vi "TSCANFD_SetData_Regs.vi"(8 "ERROR IN":errorcluster caption="错误输入（无错误）", 9 "AppName":string="LABFD", 10 "CANFD_Config_Regs":T1={"CANFD Configuration"={"Hardware Type"=8, "Hardware Subtype"=enum."TC1016", "AArbRateKbps"=250.0, "AListenOnly"=enum."Normal", "Int120Ohm"=enum."Enable", "EnableChannel"=enum."Enable", "AHwChannel"=0, "AAppChannel"=0, "ADataRateKbps"=250.0, "AControllerType"=0, "AControllerMode"=0, "AldHW"=0}, "CANFD_Sampling point"={"AArbSEG1"=0, "AArbSEG2"=0, "AArbPrescaler"=0, "AArbSJW"=0, "ADataSEG1"=0, "ADataSEG2"=0, "ADataPrescaler"=0, "ADataSJW"=0}} {"CANFD Configuration"."Hardware Type" items=["BUS_UNKNOWN_TYPE", "TS_TCP_DEVICE", "XL_USB_DEVICE", "TS_USB_DEVICE", "PEAK_USB_DEVICE", "KVASER_USB_DEVICE", "ZLG_USB_DEVICE", "ICS_USB_DEVICE", "TS_TC1005_DEVICE", "CANABLE_USB_DEVICE", "TS_WIRELESS_OBD", "TS_USB_DEVICE_EX", "IXXAT_USB_DEVICE", "TS_ETH_IF_DEVICE", "TS_USB_IF_DEVICE", "BUS_DEV_TYPE_COUNT"]; "CANFD Configuration"."AHwChannel" items=["CHN1", "CHN2", "CHN3", "CHN4", "CHN5", "CHN6", "CHN7", "CHN8", "CHN9", "CHN10", "CHN11", "CHN12", "CHN13", "CHN14", "CHN15", "CHN16", "CHN17", "CHN18", "CHN19", "CHN20", "CHN21", "CHN22", "CHN23", "CHN24", "CHN25", "CHN26", "CHN27", "CHN28", "CHN29", "CHN30", "CHN31", "CHN32"]; "CANFD Configuration"."AAppChannel" items=["CHN1", "CHN2", "CHN3", "CHN4", "CHN5", "CHN6", "CHN7", "CHN8", "CHN9", "CHN10", "CHN11", "CHN12", "CHN13", "CHN14", "CHN15", "CHN16", "CHN17", "CHN18", "CHN19", "CHN20", "CHN21", "CHN22", "CHN23", "CHN24", "CHN25", "CHN26", "CHN27", "CHN28", "CHN29", "CHN30", "CHN31", "CHN32"]; "CANFD Configuration"."AControllerType" items=["lfdtCAN", "lfdtISOFDCAN", "lfdtNonISOFDFDCAN"]; "CANFD Configuration"."AControllerMode" items=["lfdmNormal", "lfdmACKOff", "lfdmRestricted"]}, 11 "PATH":path) -> (0 "ERROR OUT":errorcluster caption="错误输出", 3 "PATH OUT":path, 4 "configure_baudrate_return":i32, 6 "mapping_return":i32)   [LabVIEW 2014]
doc: "tsapp_set_mapping_verbose ：\nFunction Introduction ：\nBefore using hardware devices, map the channels (CAN/CANFD/LIN) for the application program\n(i.e. binding) specifies the designated channel of the CAN device. This operation can also be performed on\nThe device management interface of TSMaster is completed, and this part of the operation is not required in the code.\nRegarding the channel mapping function, there are still unclear areas. Please refer to the document: TsMasterApi HardwareMap.pdf\nCall location ：\nCall this function to complete the hardware binding before the application connects to the CAN tool.\ninput parameter \nAppName: Application Name: The name of the application bound to this Map, which should be consistent with the name in initialized lib_tsmaster\nagreement\nAAppChannelType: Channel type: including APP_CAN, APP_LIN AAppChannel: Channel number of the application: This is the channel number used by the upper level program\nAHardwareName: Hardware name: such as TOSUN, Vector, etc., can also be left blank, mainly for the convenience of users to view\nAHardwareType: Hardware type: According to TLIBBusToolDeviceType, it includes all mainstream CANs currently on the market\nCard hardware Among them, the definition of tool enumeration types is as follows:\npublic enum TLIBBusToolDeviceType : int {\nBUS_UNKNOWN_TYPE = 0, TS_TCP_DEVICE = 1, XL_USB_DEVICE = 2, TS_USB_DEVICE = 3, PEAK_USB_DEVICE = 4, KVASER_USB_DEVICE = 5, ZLG_USB_DEVICE = 6, ICS_USB_DEVICE = 7, TS_TC1005_DEVICE = 8\n};\nAHardwareSubType: The sub devices under this device type, such as TS-USB-Device on the same star, are included below TC1001, TL1002, TC1011 and other series of products\nAHardwareIndex: Supports inserting multiple identical hardware devices simultaneously, such as inserting two TC1001 devices at the same time. This is used to select\nIs it the channel of device 1 or device 2\nAHardwareChannel: The channel for hardware devices, for example, TC1005 has 5 hardware channels, and this parameter is used to select the appropriate one\nCorresponding hardware channels\nAEnable Mapping: Is this mapping enabled? If set to false, the channel cannot be used。\nReturn value ：\n==0: Execution successful\nOther: Query error code\n\n\ntsapp_configure_baudrate_canfd :\nFunction Name\nint tsapp_configure_baudrate_canfd( int AIdxChn, Single AArbRateKbps, Single ADataRateKbps, TLIBCANFDControllerType AControllerType, TLIBCANFDControllerMode AControllerMode, Boolean AInstallTermResistor120Ohm);\nFunction Introduction\nConfigure hardware parameters such as baud rate for CANFD channel\nCall location\nBefore connecting to the CAN tool, call this function to configure hardware device parameters\n\ninput parameter :\nAIdxChn: Application Channel\nAArbRateKbps: Arbitration field baud rate\nADataRateKbps: Data field baud rate\nACcontrollerType: Controller type, including: Classic CAN (lfdtCAN=0), ISOCANFD (lfdtISOCAN)=\n1) NoISOCANFD (lfdtNonISOCAN=2) ACntrollerMode: Controller working mode, including: normal working mode (lfdmNormal=0), disable ACK mode\n(lfdmaCKOff=1), Restricted Mode (lfdmaRestricted=2) AInstallTermResistor120Ohm: Enable internal terminal resistance\nReturn value :\n==0: Connection successful\nOther: Check for error codes"
uses:
  Utilities/Typedef/Hardware_Subtype.ctl
  Typedef/TSCAN_CANFD_Configuration.ctl
  Typedef/TSCAN_CANFD_Configuration_Regs.ctl
  All_Control/Typedef/Hardware Type.ctl
panel:
  # "用N路can通道，设置N路CAN通道"
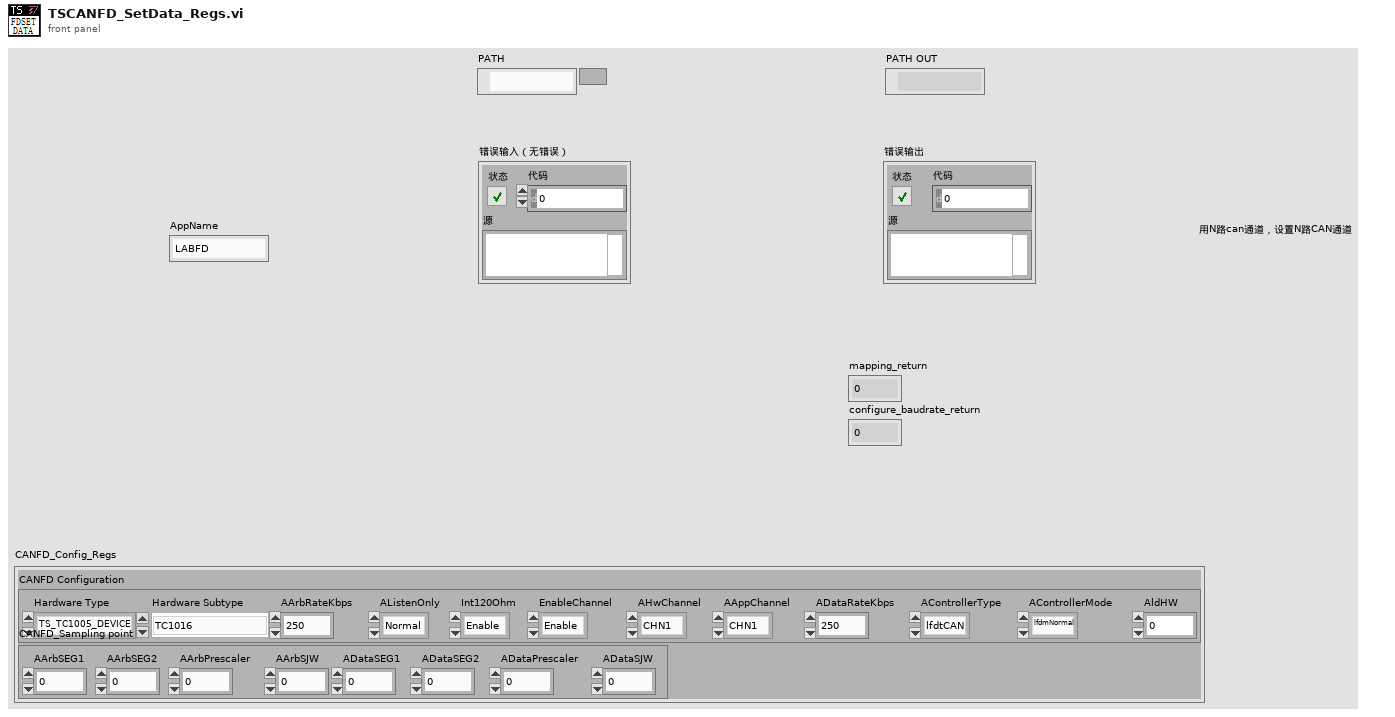
[diagram p1: front panel]
types:
  T1 = typedef "TSCAN_CANFD_Configuration_Regs.ctl" = cluster{"CANFD Configuration":T2, "CANFD_Sampling point":cluster{"AArbSEG1":i32, "AArbSEG2":i32, "AArbPrescaler":i32, "AArbSJW":i32, "ADataSEG1":i32, "ADataSEG2":i32, "ADataPrescaler":i32, "ADataSJW":i32}}
  T2 = typedef "TSCAN_CANFD_Configuration.ctl" = cluster{"Hardware Type":T3, "Hardware Subtype":T4, "AArbRateKbps":sgl, "AListenOnly":enum16{"Normal", "ListenOnly"}, "Int120Ohm":enum16{"Disable", "Enable"}, "EnableChannel":enum16{"Disable", "Enable"}, "AHwChannel":i32, "AAppChannel":i32, "ADataRateKbps":sgl, "AControllerType":i32, "AControllerMode":i32, "AldHW":i32}
  T3 = typedef "Hardware Type.ctl" = i32
  T4 = typedef "Hardware_Subtype.ctl" = enum16{"TS_UNKNOWN_DEVICE", "TSCAN_PRO", "TSCAN_Lite1", "TC1001", "TL1001", "TC1011", "TM5011", "TC1002", "TC1014", "TSCANFD2517", "TC1026", "TC1016", "TC1012", "TC1013", "TLog1002", "TC1034", "TC1018", "GW2116", "TC2115", "MP1013", "TC1113", "TC1114", "TP1013", "TC1017", "TP1018", "TF10XX", "TL1004_FD_4_LIN_2", "TE1051", "TP1051", "TP1034", "TTS9015", "TP1026", "TTS1026", "TTS1034", "TTS1018", "TL1011", "TTS1015_LiAuto", "TTS1013_LiAuto", "TTS1016Pro", "TC1054Pro", "TC1054", "TLog1038", "TO1013", "TC1034Pro", "TC1018Pro", "TC1038Pro", "TS_DEV_END"}
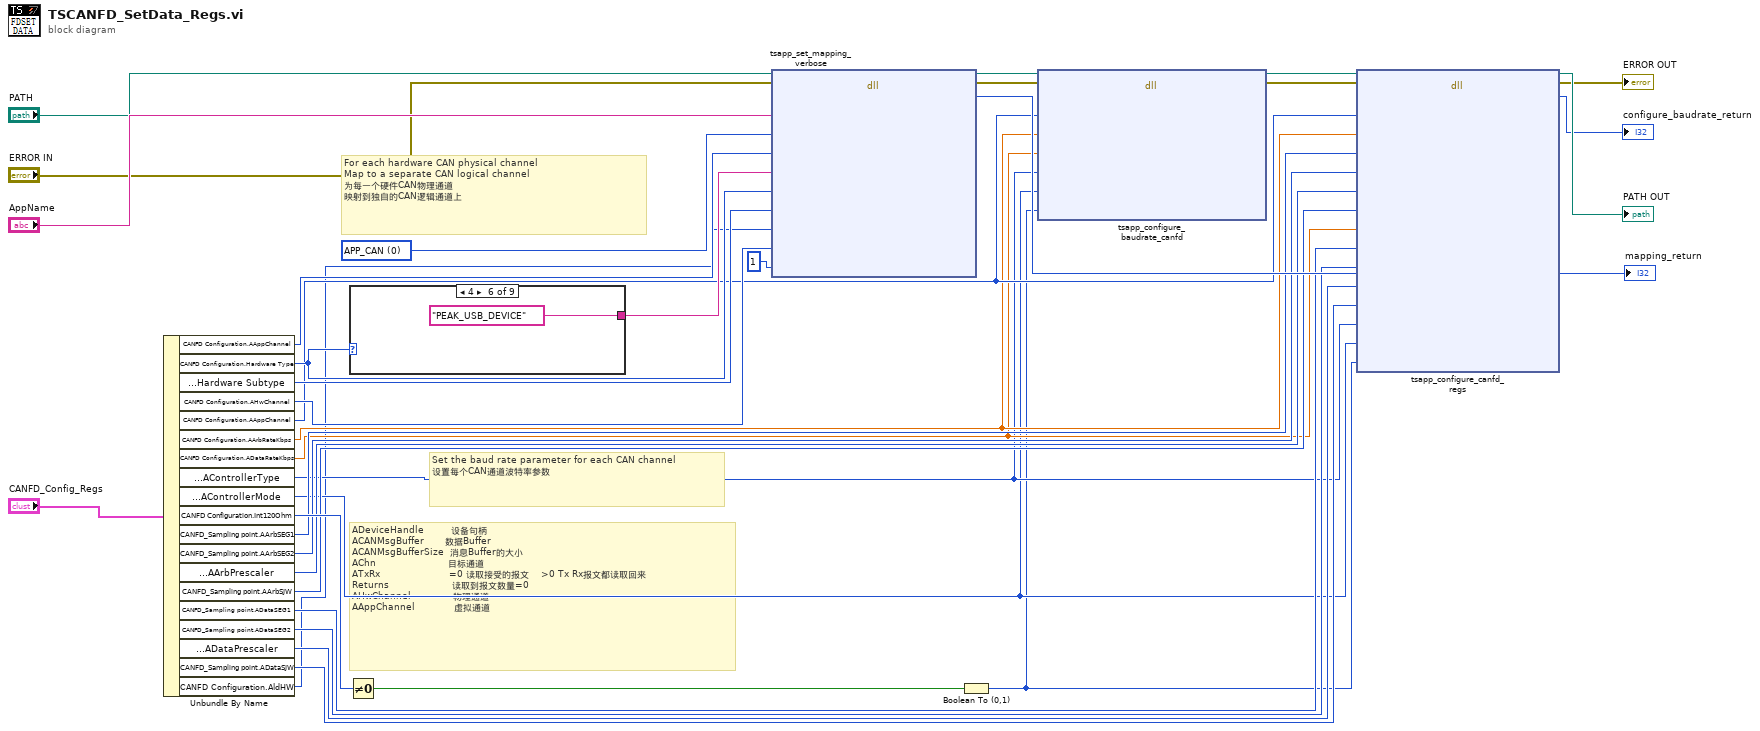
[diagram p0: block diagram]
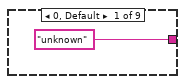
[diagram p2: hidden frame]
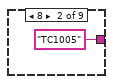
[diagram p3: hidden frame]
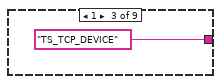
[diagram p4: hidden frame]
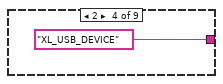
[diagram p5: hidden frame]
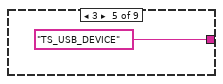
[diagram p6: hidden frame]
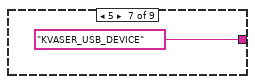
[diagram p7: hidden frame]
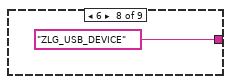
[diagram p8: hidden frame]
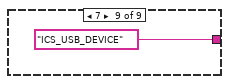
[diagram p9: hidden frame]
diagram:
  w35 = 0 items=["APP_CAN", "APP_LIN"] ("AAppChannelType")
  # "ADeviceHandle         设备句柄\nACANMsgBuffer       数据Buffer\nACANMsgBufferSize  消息Buffer的大小\nAChn                        目标通道\nATxRx                       =0 读取接受的报文    >0 Tx Rx报文都读取回来\nReturns                     读取到报文数量=0\nAHwChannel              物理通道\nAAppChannel             虚拟通道"
  # "Set the baud rate parameter for each CAN channel\n设置每个CAN通道波特率参数"
  # "For each hardware CAN physical channel\nMap to a separate CAN logical channel\n为每一个硬件CAN物理通道\n映射到独自的CAN逻辑通道上"
  n1 = Unbundle By Name("CANFD_Config_Regs") -> ("CANFD Configuration.AAppChannel"=w34:i32, "CANFD Configuration.Hardware Type"=w32:T3, "CANFD Configuration.Hardware Subtype"=w31:T4, "CANFD Configuration.AHwChannel"=w30:i32, "CANFD Configuration.AAppChannel"=w7:i32, "CANFD Configuration.AArbRateKbps"=w6:sgl, "CANFD Configuration.ADataRateKbps"=w5:sgl, "CANFD Configuration.AControllerType"=w4:i32, "CANFD Configuration.AControllerMode"=w3:i32, "CANFD Configuration.Int120Ohm"=w27:enum16{"Disable", "Enable"}, "CANFD_Sampling point.AArbSEG1"=w19:i32, "CANFD_Sampling point.AArbSEG2"=w18:i32, "CANFD_Sampling point.AArbPrescaler"=w17:i32, "CANFD_Sampling point.AArbSJW"=w16:i32, "CANFD_Sampling point.ADataSEG1"=w15:i32, "CANFD_Sampling point.ADataSEG2"=w14:i32, "CANFD_Sampling point.ADataPrescaler"=w13:i32, "CANFD_Sampling point.ADataSJW"=w12:i32, "CANFD Configuration.AldHW"=w1:i32)
  n2 = Not Equal To 0?(x=w27) -> (x != 0?=w28:bool)
  n3 = case shown="4" w32 {
    tunnel: ["unknown" ("AHardwareName") "TC1005" ("AHardwareName") "TS_TCP_DEVICE" ("AHardwareName") "XL_USB_DEVICE" ("AHardwareName") "TS_USB_DEVICE" ("AHardwareName") "PEAK_USB_DEVICE" ("AHardwareName") "KVASER_USB_DEVICE" ("AHardwareName") "ZLG_USB_DEVICE" ("AHardwareName") "ICS_USB_DEVICE" ("AHardwareName")] -> w33
    frame 0, Default {
    }
    frame 8 {
    }
    frame 1 {
    }
    frame 2 {
    }
    frame 3 {
    }
    frame 4 {
    }
    frame 5 {
    }
    frame 6 {
    }
    frame 7 {
    }
  }
  n4 = dll-call lib="PTH2Habs CUsers\nAdministratorDesktopTS_Can通讯PathTSMaster.dll" fn="tsapp_set_mapping_verbose"(path in="PATH", error in="ERROR IN", "FAPppName"="AppName", "AChnType"=w35, "FAppChannelIndex"=w34, "AHWDeviceName"=w33, "AHWDeviceType"=w32, "AHWDeviceSubType"=w31, "AldHW"=w1, "AldHWChn"=w30, "FMappingDisabled"=u32 1) -> (path out=w11:path, error out=w9:errorcluster, "tsapp_set_mapping_verbose"=→"mapping_return":i32)  [unwired: 10 in]
  n5 = Boolean To (0,1)(Boolean=w28) -> (0, 1=w2:i16)
  n6 = dll-call lib="PTH27abs EDemo同星\nTSCAN_V1.0ConfigTSMaster.dll" fn="tsapp_configure_baudrate_canfd"(path in=w11, error in=w9, "ALdxChn"=w7, "AArbRateKbps"=w6, "ADataRateKbps"=w5, "AControllerType"=w4, "AControllerMode"=w3, "AlnstallTermResistor120Ohm"=w2) -> (path out=w10:path, error out=w8:errorcluster)  [unwired: 8 in]
  n7 = dll-call lib="C:/Users/XYY/Desktop/LabView Demo/TSCAN_LB2018_V1.3_20220301/Config/TSMaster.dll" fn="tsapp_configure_canfd_regs"(path in=w10, error in=w8, "AIdxChn"=w7, "AArbBaudrate"=w6, "AArbSEG1"=w19, "AArbSEG2"=w18, "AArbPrescaler"=w17, "AArbSJW"=w16, "ADataBaudrate"=w5, "ADataSEG1"=w15, "ADataSEG2"=w14, "ADataPrescaler"=w13, "ADataSJW"=w12, "AControllerType"=w4, "AControllerMode"=w3, "A120OhmConnected"=w2) -> (path out=→"PATH OUT":path, error out=→"ERROR OUT":errorcluster, "返回类型"=→"configure_baudrate_return":i32)  [unwired: 15 in]
